vi "DPO_7K_Set_Horizontal_Scale.vi"(8 "Error In":errorcluster, 9 "Epoch":dbl format="%#_6ps", 10 "Sampling Frequency":u16(ring) items=["3.125 Sa/s", "5 Sa/s", "6.25 Sa/s", "7.8125 Sa/s", "10 Sa/s", "12.5 Sa/s", "15.625 Sa/s", "20 Sa/s", "25 Sa/s", "31.25 Sa/s", "50 Sa/s", "62.5 Sa/s", "78.125 Sa/s", "100 Sa/s", "125 Sa/s", "156.25 Sa/s", "200 Sa/s", "250 Sa/s", "312.5 Sa/s", "390.625 Sa/s", "400 Sa/s", "500 Sa/s", "625 Sa/s", "781.25 Sa/s", "1 kSa/s", "1.25 kSa/s", "1.5625 kSa/s", "2 kSa/s", "2.5 kSa/s", "3.125 kSa/s", "3.90625 kSa/s", "4 kSa/s", "5 kSa/s", "6.25 kSa/s", "7.8125 kSa/s", "10 kSa/s", "12.5 kSa/s", "15.625 kSa/s", "20 kSa/s", "25 kSa/s", "31.25 kSa/s", "39.0625 kSa/s", "50 kSa/s", "62.5 kSa/s", "78.125 kSa/s", "100 kSa/s", "125 kSa/s", "156.25 kSa/s", "200 kSa/s", "244.14063 kSa/s", "250 kSa/s", "312.5 kSa/s", "390.625 kSa/s", "500 kSa/s", "625 kSa/s", "781.25 kSa/s", "1 MSa/s", "1.2207 MSa/s", "1.25 MSa/s", "1.5625 MSa/s", "1.95313 MSa/s", "2.44141 MSa/s", "2.5 MSa/s", "3.125 MSa/s", "3.90625 MSa/s", "4.88281 MSa/s", "5 MSa/s", "6.25 MSa/s", "7.8125 MSa/s", "9.76563 MSa/s", "12.5 MSa/s", "1.5625 MSa/s", "25 MSa/s", "31.25 MSa/s", "39.0625 MSa/s", "62.5 MSa/s", "78.125 MSa/s", "125 MSa/s", "156.25 MSa/s", "250 MSa/s", "312.5 MSa/s", "625 MSa/s", "781.25 MSa/s", "1.25 GSa/s", "1.5625 GSa/s", "3.125 GSa/s", "6.25 GSa/s", "12.5 GSa/s", "25 GSa/s", "50 GSa/s", "100 GSa/s", "200 GSa/s (ATI only)"], 11 "VISA resource name in":refnum<visa-resource-name>) -> (0 "Error Out":errorcluster, 3 "VISA resource name out":refnum<visa-resource-name>)   [LabVIEW 2020]
uses:
  subVI/Return_To_Interface.ctl
  subVI/Set_Configuration.ctl
panel:
  in  "Set":T1
  in  "Return to Interface":T2
  out "output string":string
  # "SET HORIZONTAL SCALE"
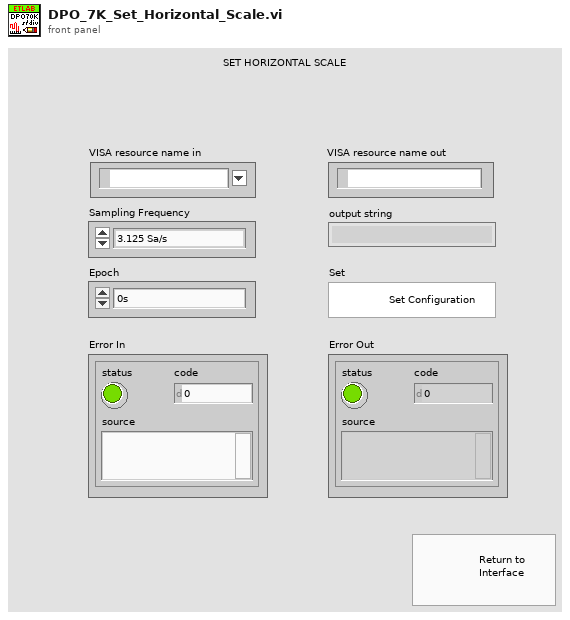
[diagram p1: front panel]
types:
  T1 = typedef "Set_Configuration.ctl" = bool
  T2 = typedef "Return_To_Interface.ctl" = bool
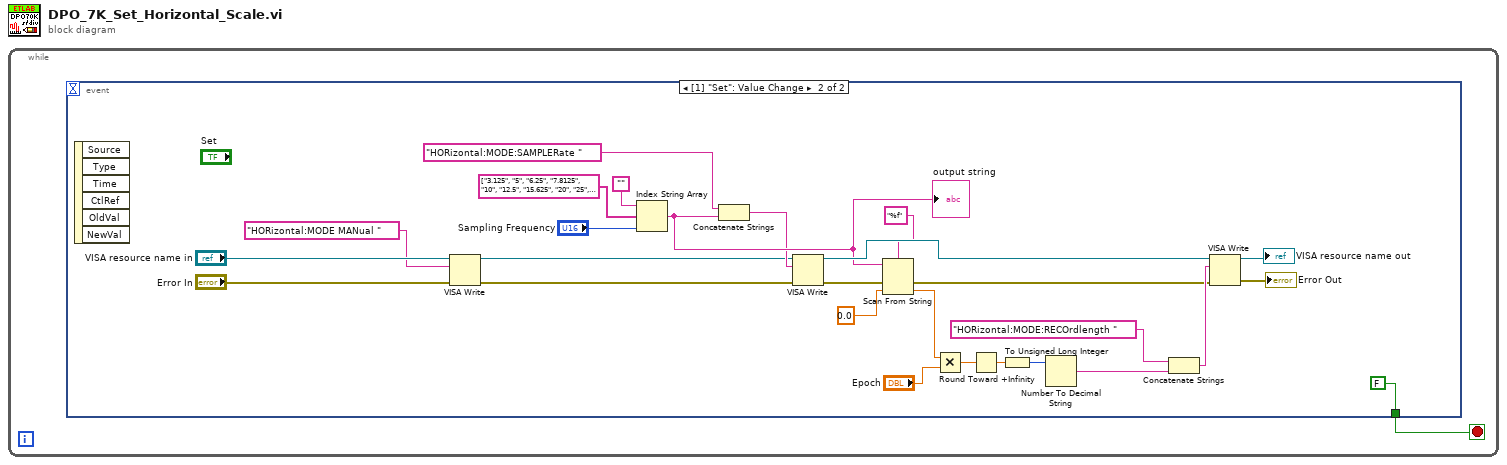
[diagram p0: block diagram]
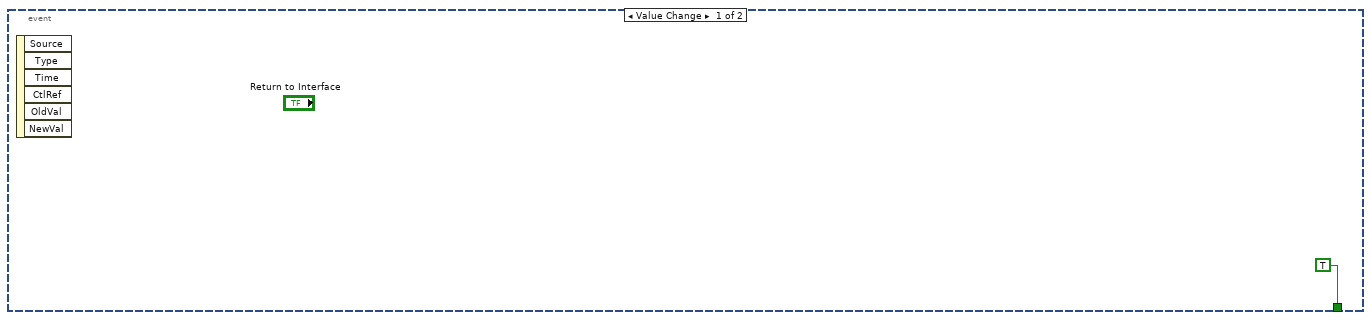
[diagram p2: hidden frame]
diagram:
  n1 = while {
    stop <- w1 stop-if-true
    n2 = event shown="[1] \"Set\": Value Change" {
      selector: _ -> [_ _]
      dyn-events: _ -> [_ _]
      timeout: _ -> [_ _]
      tunnel: [TRUE FALSE] -> w1
      event Value Change {
        n3 = event-data() -> ()  [unwired: 1 in, 6 out]
      }
      event Value Change {
        n4 = event-data() -> ()  [unwired: 1 in, 6 out]
        n5 = VISA Write(VISA resource name="VISA resource name in", write buffer="HORizontal:MODE MANual ", error in (no error)="Error In") -> (VISA resource name out=w14:refnum<visa-resource-name>, error out=w15:errorcluster)  [unwired: 1 out]
        n6 = Index String Array(1:"Sampling Frequency", 2:string[] ["3.125", "5", "6.25", "7.8125", "10", "12.5", "15.625", "20", "25", "31.25", "50", "62.5", "78.125", "100", "125", "156.25", "200", "250", "312.5", "390.625", "400", "500", "625", "781.25", "1e3", "1.25e3", "1.5625e3", "2e3", "2.5e3", "3.125e3", "3.90625e3", "4e3", "5e3", "6.25e3", "7.8125e3", "10e3", "12.5e3", "15.625e3", "20e3", "25e3", "31.25e3", "39.0625e3", "50e3", "62.5e3", "78.125e3", "100e3", "125e3", "156.25e3", "200e3", "244.14063e3", "250e3", "312.5e3", "390.625e3", "500e3", "625e3", "781.25e3", "1e6", "1.2207e6", "1.25e6", "1.5625e6", "1.95313e6", "2.44141e6", "2.5e6", "3.125e6", "3.90625e6", "4.88281e6", "5e6", "6.25e6", "7.8125e6", "9.76563e6", "12.5e6", "1.5625e6", "25e6", "31.25e6", "39.0625e6", "62.5e6", "78.125e6", "125e6", "156.25e6", "250e6", "312.5e6", "625e6", "781.25e6", "1.25e9", "1.5625e9", "3.125e9", "6.25e9", "12.5e9", "25e9", "50e9", "100e9", "200e9"] ("Frequencies"), 3:"") -> (0:w17:string)
        "output string" <- w17
        n7 = Concatenate Strings("HORizontal:MODE:SAMPLERate ", w17) -> (w16:string)
        n8 = VISA Write(VISA resource name=w14, write buffer=w16, error in (no error)=w15) -> (VISA resource name out=w26:refnum<visa-resource-name>, error out=w18:errorcluster)  [unwired: 1 out]
        n9 = Scan From String(format string="%f", input string=w17, error in=w18, default 1=0.0 ("default value 1")) -> (error out=w25:errorcluster, output 1=w19:dbl)  [unwired: 1 in, 2 out]
        n10 = Multiply(x=w19, y="Epoch") -> (x*y=w21:dbl)
        n11 = Round Toward +Infinity(x=w21) -> (ceil(x): smallest int >= x=w22:dbl)
        n12 = To Unsigned Long Integer(number=w22) -> (unsigned 32bit integer=w23:u32)
        n13 = Number To Decimal String(number=w23) -> (decimal integer string=w24:string)  [unwired: 1 in]
        n14 = Concatenate Strings("HORizontal:MODE:RECOrdlength ", w24) -> (w27:string)
        n15 = VISA Write(VISA resource name=w26, write buffer=w27, error in (no error)=w25) -> (VISA resource name out=→"VISA resource name out":refnum<visa-resource-name>, error out=→"Error Out":errorcluster)  [unwired: 1 out]
      }
    }
  }
